vi "reg_visu OPC.vi"(7 "name":string="GM10", 9 "stop":bool, 10 "connect (T)":bool=TRUE) -> (0 "error out":errorcluster, 5 "This VI":refnum<vi>)   [LabVIEW 2019]
uses:
  Heating/ctl/Z_OnSwitch/Z_OnSwitch.xctl
  Heating/ctl/Z_ind_heating.ctl
  Heating/ctl/Z_Hswitch/Z_Hswitch.xctl
  ctl/Y/Y.xctl
  Heating/ctl/Z_State.ctl
  Heating/ctl/Y_state.ctl
  <vilib>/OPCUA/controls/OPC UA StatusCode.ctl
  Heating/ctl/ZY_state.ctl
  Heating/ctl/Z.ctl
  Heating/ctl/Y_source.ctl
  Heating/ctl/ZM_State.ctl
  Heating/ctl/Y.ctl
  Inputs/Ctl/Parameter State.ctl
  Alarms/Ctl/ALR_Status.ctl
  Heating/ctl/ZY_state_OPC.ctl
  <vilib>/OPCUA/controls/Write Variant Request.ctl
  <vilib>/OPCUA/controls/NodeId.ctl
  <vilib>/OPCUA/controls/Write Status.ctl
  08a30d42-25e3-4a58-beca-1d562a75ea40.vi
  fbc51cc2-a17d-4d51-90ca-ef1d5e9adb43.vi
  81bac83f-5a8a-4521-9bb9-45d0222ee4c6.vi
  3276b797-77fd-4487-96b2-8bfe15282525.vi
  45230f51-ed9d-4592-a49a-e0edfe92ddd1.vi
  <vilib>/NI/AMC/Read Termination Message.vi
  <vilib>/NI/AMC/Create Single Message.vi
  <vilib>/NI/AMC/Update Message Routing Info.vi
  Counter/Generator simplified.vi
  <vilib>/NI/AMC/Globals.vi
  <vilib>/NI/AMC/Send Message.vi
  Heating/Global stop.vi
  <vilib>/OPCUA/client/Multiple Read String.vi
  <vilib>/JDP Science/JSONtext/JSON text to Variant.vi
  <vilib>/OPCUA/client/Multiple Write Variant.vi
  Heating/Heating.lvlib
  <vilib>/OPCUA/NI OPC UA Client.lvlib
  OPC/OPC addons.lvlib
  Inputs/Inputs.lvlib
  <vilib>/NI/AMC/AMC.lvlib
  Alarms/Alarms.lvlib
panel:
  out "PV":dbl(slide) scale=0.0..10.0
  in  "Scale max":dbl=1.0 format="%#_13g"
  in  "name 4":string="Осн."
  in  "Unit":enum16{"l/h", "m3/h"}(ring)
  in  "name 3":string="Осн."
  in  "t":dbl=10.5 caption="сек."
  in  "alarm val":dbl=3.01 caption="m3/h"
  in  "auto":dbl=15.888 caption="Зависимый"
  in  "k":dbl=1.459 caption="Коэфф"
  in  "Y_SP":cluster{dbl, dbl, dbl}(xcontrol)
  in  "message name":string="AI redefine"
  out "status":string
  in  "process":bool
  in  "state variables":cluster{"CurrentFile":path}
  in  "security policy":T1
  out "JSON string":string
  in  "JSON":string
  in  "Write controls":bool
  out "T stage":dbl format="%<%M:%S>t"
  in  "ALRL1_reset":bool
  in  "ALRL2_reset":bool
  out "Z3 ind":T2
  in  "Z_OnSwitch":bool(xcontrol)
  in  "Z_Hswitch":bool(xcontrol)
  out "Z5 State":string
  # "Время установки"
  # "Аварийный"
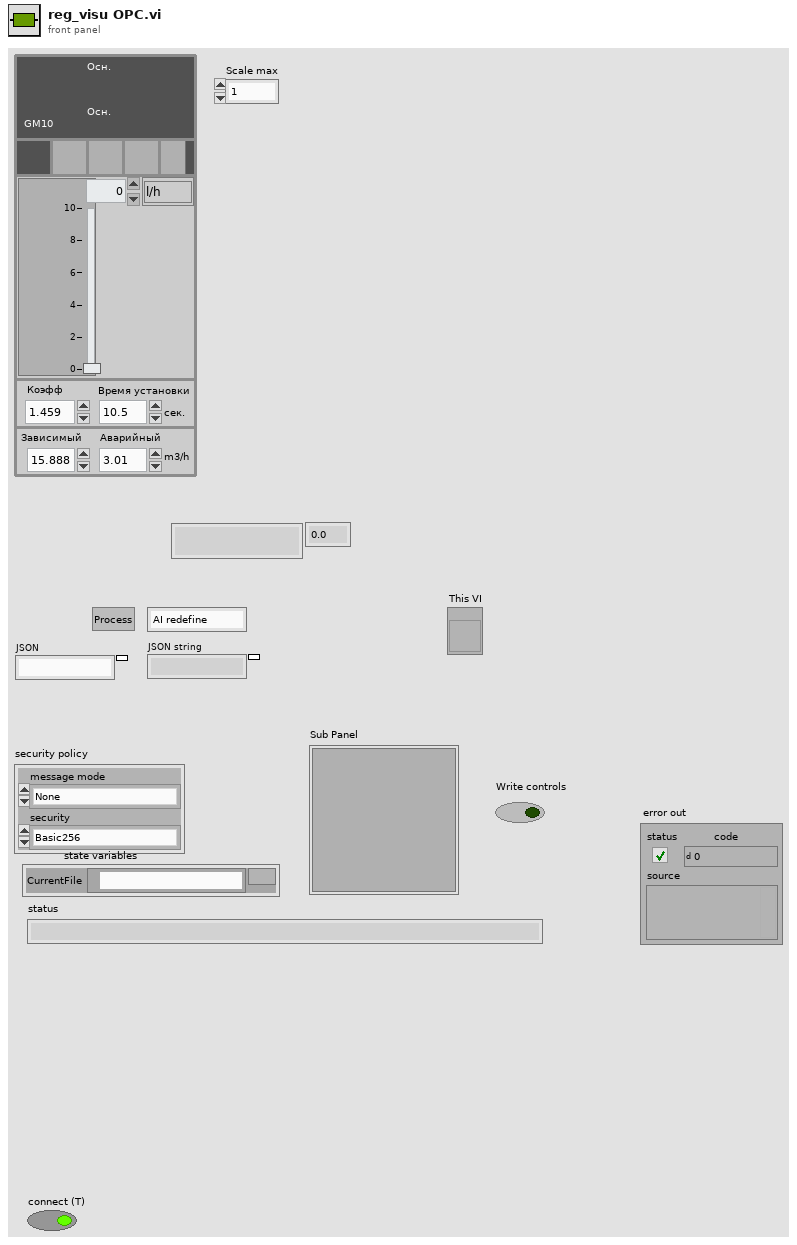
[diagram p1: front panel]
types:
  T1 = cluster{"message mode":enum16{"None", "Sign", "Sign and Encrypt"}, "security":enum16{"Basic256", "Basic128Rsa15"}}
  T2 = typedef "Heating.lvlib/Z_ind_heating.ctl" = u16
  T3 = typedef "AMC.lvlib/Message Queue.ctl" = refnum<queue>
  T4 = typedef "Write Variant Request.ctl" = cluster{"node ID":T5, "value":variant, "timestamp (current time)":timestamp, "node status":T6}
  T5 = typedef "NodeId.ctl" = string
  T6 = typedef "Write Status.ctl" = u32
  T7 = typedef "OPC UA Client Refnum.ctl" = refnum<k21>
  T8 = typedef "Subscription ID.ctl" = u32
  T9 = typedef "Heating.lvlib/Y_source.ctl" = enum8{"initialize", "local disabled", "local hand", "hand", "auto", "dist"}
  T10 = cluster{"connect":bool, "SP_Source":T9, "SP_Set":dbl, "SP":dbl}
  T11 = typedef "Heating.lvlib/Z_State.ctl" = enum8{"initialization", "alarm", "disabled", "not ready", "stop ready", "reserv", "switched off", "reserv2", "switched on", "check", "on min", "decrease out", "on", "increase out", "on max"}
  T12 = cluster{"connect":bool, "Z_Source":T9, "Z_State_heating":T11}
  T13 = typedef "Heating.lvlib/ZM_State.ctl" = enum8{"initialization", "stop", "start_cmd", "contactor_on_cmd", "heating", "on", "stop_cmd", "power_down", "contactor_off_cmd", "cooling", "restart_delay"}
  T14 = typedef "Heating.lvlib/ZY_state_OPC.ctl" = cluster{"Z":cluster{"Z_Source":u8, "Z_SetState":u8, "Z_State":u8, "Z_State_T":u32, "ZM_State":u8, "ZM_State_T":u32, "ALR  L1":bool, "ALR  L2":bool, "HH_run":i32}, "Y":cluster{"Y_Source":u8, "Y_SetState":u8, "SP_Set":dbl, "SP":dbl, "PV":dbl, "Y":dbl, "Y_State":cluster{"code":i32, "visible":bool, "color":u32}, "YB":bool}, "ALR_Status":cluster{"status":bool, "code":i32, "level":i32}[]}
  T15 = cluster{"Z_HSw":u32, "Z_HSetState":u32, "Y_HSw":u32, "Y_HSetState":u32, "SP":dbl, "Y_H":dbl, "Reset_ALR":bool}
  T16 = typedef "Heating.lvlib/Y_state.ctl" = enum8{"initialize", "alarm", "min", "stop", "hand", "auto", "max"}
  T17 = typedef "Heating.lvlib/ZY_state.ctl" = cluster{"Z":T18, "Y":T19, "ALR_Status":T21[]}
  T18 = typedef "Heating.lvlib/Z.ctl" = cluster{"Z_Source":T9, "Z_SetState":T11, "Z_State":T11, "Z_State_T":u32, "ZM_State":T13, "ZM_State_T":u32, "ALR  L1":bool, "ALR  L2":bool, "HH_run":i32}
  T19 = typedef "Heating.lvlib/Y.ctl" = cluster{"Y_Source":T9, "Y_SetState":T16, "SP_Set":dbl, "SP":dbl, "PV":dbl, "Y":dbl, "Y_State":T20, "YB":bool}
  T20 = typedef "Inputs.lvlib/Parameter State.ctl" = cluster{"code":i32, "visible":bool, "color":u32, "source":string}
  T21 = typedef "Alarms.lvlib/ALR_Status.ctl" = cluster{"status":bool, "code":i32, "level":i32, "source":string}
  T22 = typedef "OPC UA StatusCode.ctl" = u32
  T23 = enum32{"Invalid Status", "Unconnected", "Active", "Idle", "Error", "Connecting"}
  T24 = cluster{"node ID":T5, "value ":string, "timestamp":timestamp, "status":T22}[]
  T25 = typedef "LVDataSocketStatusTypeDef.ctl" = cluster{"Code":enum32{"Invalid Status", "Unconnected", "Active", "Idle", "Error", "Connecting"}, "Text":string}
  T26 = cluster{"node ID":T5, "value ":string, "timestamp":timestamp, "status":T22}
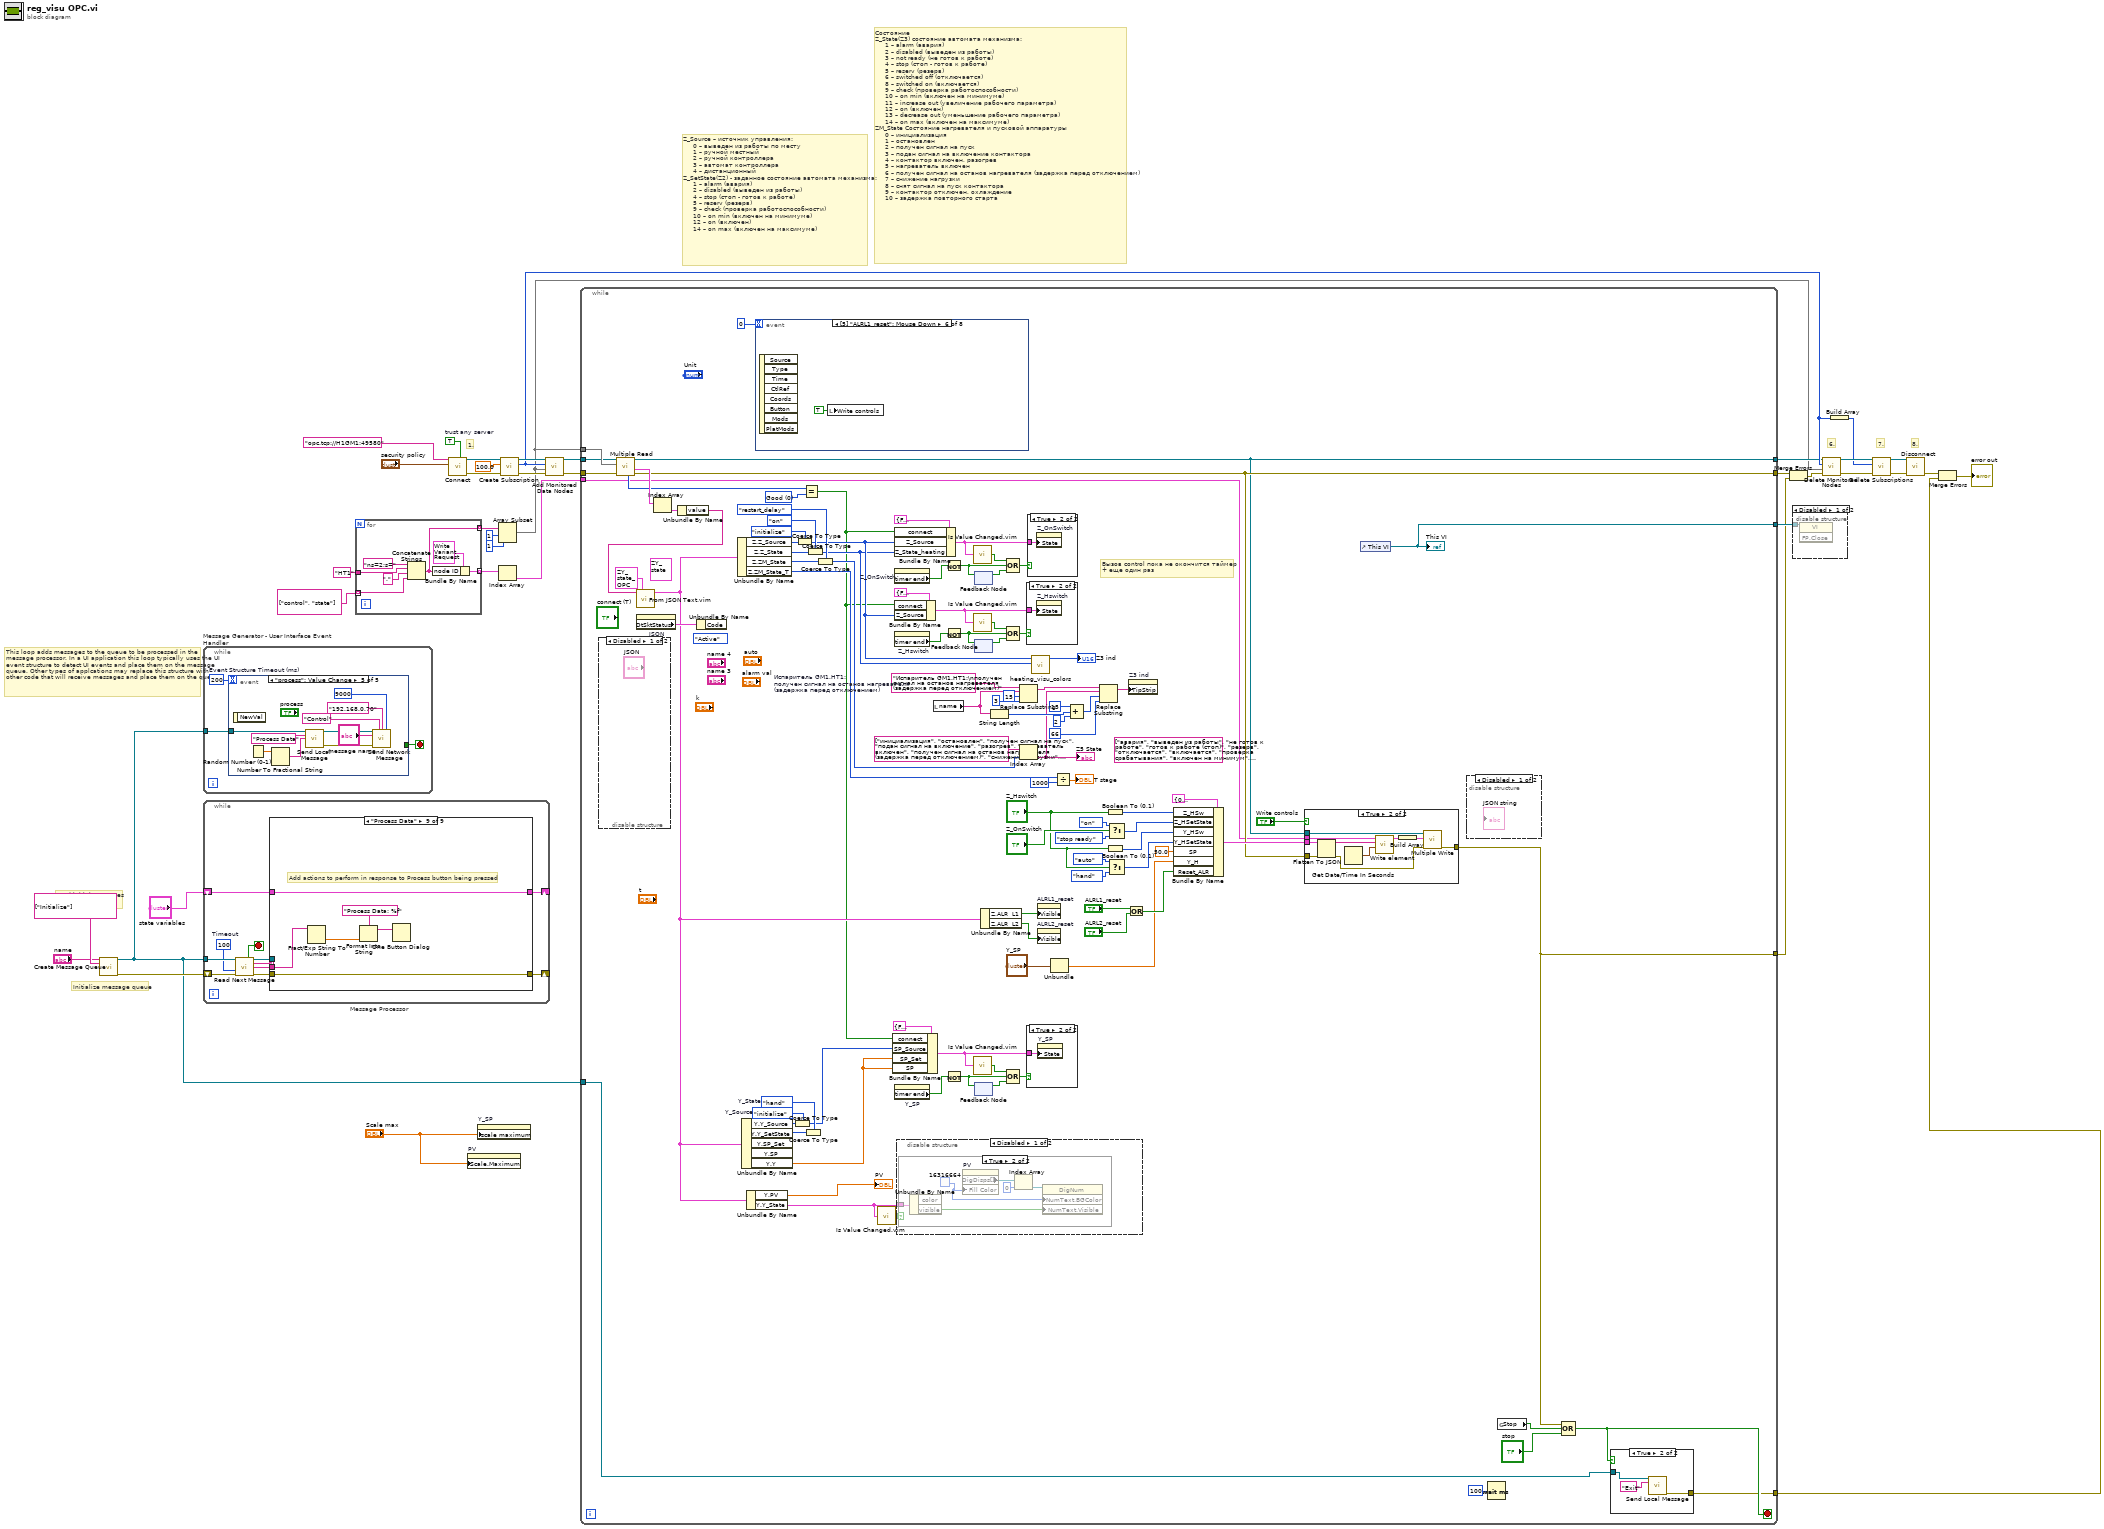
[diagram p0: block diagram]
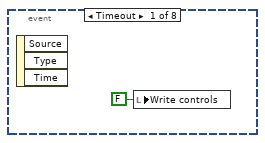
[diagram p9: hidden frame]
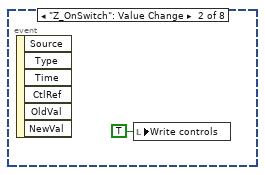
[diagram p10: hidden frame]
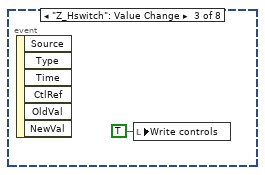
[diagram p11: hidden frame]
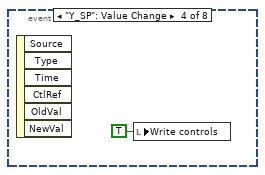
[diagram p12: hidden frame]
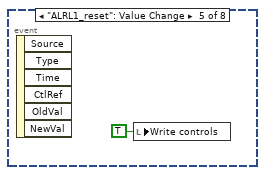
[diagram p13: hidden frame]
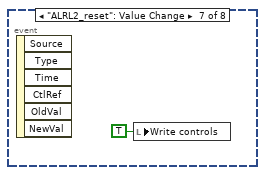
[diagram p14: hidden frame]
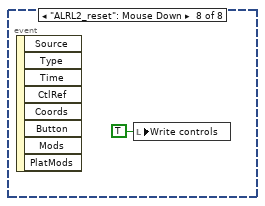
[diagram p15: hidden frame]
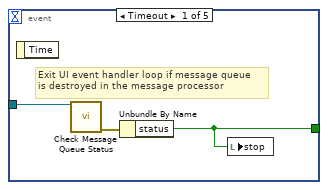
[diagram p19: hidden frame]
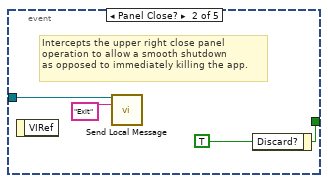
[diagram p20: hidden frame]
diagram:
  w31 = TRUE  # trust any server
  # "This loop adds messages to the queue to be processed in the message processor. In a UI application this loop typically uses the UI event structure to detect UI events and place them on the message queue. Other types of applcations may replace this structure with other code that will receive messages and place them on the queue."
  # "Initialize message queue"
  # "Load initial messages\non the queue"
  # "7."
  # "8."
  # "6."
  # "1."
  # "Состояние\nZ_State(Z3) состояние автомата механизма:\n     1 – alarm (авария)\n     2 – disabled (выведен из работы)\n     3 – not ready (не готов к работе)\n     4 – stop (стоп - готов к работе)\n     5 – reserv (резерв)\n     6 – switched off (отключается)\n     8 – switched on (включается)\n     9 – check (проверка работоспособности)\n     10 – on min (включен на минимуме)\n     11 – increase out (увеличение рабочего параметра)\n     12 – on (включен)\n     13 – decrease out (уменьшение рабочего параметра)\n     14 – on max (включен на максимуме)\nZM_State Состояние нагревателя и пусковой аппаратуры\n     0 – инициализация\n     1 – остановлен\n     2 – получен сигнал на пуск\n     3 – подан сигнал на включение контактора\n     4 – контактор включен, разогрев\n     5 – нагреватель включен\n     6 – получен сигнал на останов нагревателя (задержка перед отключением)\n     7 – снижение нагрузки\n     8 – снят сигнал на пуск контактора\n     9 – контактор отключен, охлаждение\n     10 – задержка повторного старта"
  # "Z_Source – источник управления:\n     0 – выведен из работы по месту\n     1 – ручной местный\n     2 – ручной контроллера\n     3 – автомат контроллера\n     4 – дистанционный\nZ_SetState(Z2) - заданное состояние автомата механизма:\n     1 – alarm (авария)\n     2 – disabled (выведен из работы)\n     4 – stop (стоп - готов к работе)\n     5 – reserv (резерв)\n     9 – check (проверка работоспособности)\n     10 – on min (включен на минимуме)\n     12 – on (включен)\n     14 – on max (включен на максимуме)"
  n1 = call <vilib>:"Create Message Queue.vi"("message queue name"="name", "initial message names"=string[] ["Initialize"]) -> ("message queue out"=w6:T3, "error out"=w8:errorcluster)  [unwired: 12 in]
  n2 = while "Message Generator - User Interface Event Handler" {
    tunnel: w6 -> [w39]
    stop <- w40 stop-if-true
    w41 = 200  # Event Structure Timeout (ms)
    n3 = event shown="[4] \"process\": Value Change" {
      selector: _ -> [_ _ _ _ _]
      dyn-events: _ -> [_ _ _ _ _]
      timeout: w41 -> [_ _ _ _ _]
      tunnel: [w42 w47 TRUE ("Discard?") _ _] -> w40
      tunnel: w39 -> [w43 w45 w48 w51 w62]
      event Timeout {
        # "Exit UI event handler loop if message queue\nis destroyed in the message processor"
        n4 = event-data() -> ()  [unwired: 2 out]
        n5 = call <vilib>:"Check Message Queue Status.vi"("message queue in"=w43) -> ("error out"=w44:errorcluster)  [unwired: 10 in, 4 out]
        n6 = Unbundle By Name(w44) -> ("status"=w42:bool)
        n7 = local write "stop"(w42) -> ()
      }
      event Panel Close? {
        w47 = TRUE ("Discard?")
        # "Intercepts the upper right close panel\noperation to allow a smooth shutdown\nas opposed to immediately killing the app."
        n8 = event-data() -> ()  [unwired: 2 out]
        n9 = call <vilib>:"Send Local Message.vi"("message queue in"=w45, "message name"="Exit") -> ()  [unwired: 11 in, 3 out]
        n10 = event-data("Discard?"=w47) -> ()  [unwired: 1 in, 1 out]
      }
      event "stop": Value Change {
        # "Exit the application\n>> Stop this message generator loop"
        n11 = event-data() -> ()  [unwired: 7 out]
        n12 = call <vilib>:"Send Local Message.vi"("message queue in"=w48, "message name"="Exit") -> ()  [unwired: 11 in, 3 out]
      }
      event Menu Selection (User) {
        # "Add run-time menu items to the message\nqueue. The message handler case names must match the menu ItemTag names."
        n13 = event-data() -> ("ItemTag"=w52:string)  [unwired: 1 out]
        n14 = call <vilib>:"Send Local Message.vi"("message queue in"=w51, "message name"=w52) -> ()  [unwired: 11 in, 3 out]
      }
      event "process": Value Change {
        n15 = event-data() -> ()  [unwired: 2 out]
        n16 = Random Number (0-1)() -> (number: 0 to 1=w59:dbl)
        n17 = Number To Fractional String(number=w59) -> (F-format string=w60:string)  [unwired: 3 out]
        n18 = call <vilib>:"Send Local Message.vi"("message queue in"=w62, "message name"="Process Data", "message value"=w60) -> ("message queue out"=w58:T3, "error out"=w54:errorcluster)  [unwired: 10 in, 1 out]
        n19 = call <vilib>:"Send Network Message.vi"("message queue in"=w58, "receiver process"="Control", "receiver host"="192.168.0.70", "receiver port (0)"=u16 9000, "message name"="message name", "error in"=w54) -> ()  [unwired: 7 in, 3 out]
      }
    }
  }
  n20 = while "Message Processor" {
    shift-left: w8 -> [w67]
    shift-right: [w71] -> _
    tunnel: w6 -> [w68]
    shift-left: "state variables" -> [w73]
    shift-right: [w72] -> _
    stop <- w70 stop-if-true
    w63 = 100  # Timeout
    n21 = call <vilib>:"Read Next Message.vi"("message queue in"=w68, "timeout (1 ms)"=w63, "error in"=w67) -> ("exit process?"=w70:bool, "message queue out"=w69:T3, "message name"=w65:string, "message value"=w64:string, "error out"=w66:errorcluster)  [unwired: 5 in, 3 out]
    n22 = case shown="\"Process Data\"" w65 {
      selector: w65 -> [_ _ w85 _ _ _ _ _ _]
      tunnel: [w75 w82 w87 w92 w94 w96 w101 w103 w108] -> w72
      tunnel: w73 -> [w75 w82 w87 w92 w94 w96 w101 w103 w108]
      tunnel: w69 -> [_ _ _ w90 _ _ w98 _ _]
      tunnel: w66 -> [w74 w81 w86 w88 w93 w95 w99 w102 w109]
      tunnel: [w74 w81 w86 errorcluster {"status"=FALSE, "code"=0, "source"=""} ("error out") w93 w95 w97 w102 w109] -> w71
      tunnel: w64 -> [_ _ _ _ _ _ _ _ w107]
      frame "---------- Framework Operations ----------" {
        # "Dummy case to add a seperator in the Case Structure menu"
      }
      frame "", "Idle" {
        # "Update the front panel"
        # "Idle Case - this case is called after a Timeout on the Get Next Message from Queue VI, if no new messages are present on the queue. This case can be used for housekeeping tasks such as updating the UI."
        n23 = Get Date/Time String(want seconds? (F)=TRUE) -> (date string=w80:string, time string=w79:string)  [unwired: 2 out]
        n24 = Concatenate Strings(w80, " " ("string"), w79) -> (→"status":string)
      }
      frame "Missing Message Handler", Default {
        # "Call this case if a message is received that is not handled \nby any other case. Typically this is a programming error\nas a result of a typo or unhandled message/missing message handler."
        n25 = Format Into String(format string="DevError: Missing message handler for '%s\" message." ("message"), w85) -> (resulting string=w83:string)  [unwired: 2 in, 1 out]
        n26 = One Button Dialog(message=w83) -> ()  [unwired: 2 out]
      }
      frame "Error" {
        # "Proceed to Exit - Remove this if it is\nnot appropriate for the General Error case"
        # "General Error Case - this case is called if an error is passed using the error cluster below. Typically most new errors should be handed in each individual case and not passed in the rror cluster. If necessary a custom error handler case should be added and called from other cases."
        n27 = call <vilib>:"Simple Error Handler.vi"("error in (no error)"=w88) -> ()  [unwired: 1 in, 8 out]
        n28 = call <vilib>:"Send Local Message.vi"("message queue in"=w90, "message name"="Exit") -> ()  [unwired: 11 in, 3 out]
      }
      frame "---------- Generic Operations ----------" {
        # "Dummy case to add a seperator in the Case Structure menu"
      }
      frame "Initialize" {
        # "Initialize the state variables and user interface"
      }
      frame "Exit" {
        # "Destroy message queue >> this will halt the UI event handler loop"
        # "Stop the VI\n>> Perform any cleanup tasks in this message case.\n>> Clear display before closing."
        n29 = call <vilib>:"Destroy Message Queue.vi"("message queue in"=w98, "error in"=w99) -> ("error out"=w97:errorcluster)  [unwired: 11 in, 2 out]
        n30 = local write "status"("" ("Status")) -> ()
      }
      frame "---------- Application Operations ----------" {
        # "Dummy case to add a seperator in the Case Structure menu"
      }
      frame "Process Data" {
        # "Add actions to perform in response to Process button being pressed"
        n31 = Fract/Exp String To Number(string=w107) -> (number=w106:dbl)  [unwired: 4 out]
        n32 = Format Into String(format string="Process Data: %f" ("message"), w106) -> (resulting string=w104:string)  [unwired: 2 in, 1 out]
        n33 = One Button Dialog(message=w104) -> ()  [unwired: 2 out]
      }
    }
  }
  n34 = for {
    tunnel: string[] ["control", "state"] -> [w110] mode=indexing
    tunnel: "HT1" ("Folder Name") -> [w116]
    tunnel: [w113] -> w20 mode=indexing
    tunnel: [w112] -> w16 mode=indexing
    n35 = Concatenate Strings("ns=2;s=" ("string"), w116, "." ("string"), w110) -> (w113:string)
    n36 = Bundle By Name(cluster=T4 {"node ID"="", "value"=variant, "timestamp (current time)"=timestamp(0 s since 1904-01-01), "node status"=0} ("request"), "node ID"=w113) -> (w112:T4)
  }
  n37 = call <vilib>:"Connect.vi"("trust any server (F)"=w31, "security policy"="security policy", "server endpoint URL"="opc.tcp://H1GM1:49580" ("server endpoint URL 2")) -> ("error out"=w34:errorcluster, "OPC UA client refnum out"=w35:T7)  [unwired: 6 in, 1 out]
  n38 = property on="PV" class="Slide (strict)"("Scale.Maximum"="Scale max") -> ()  [unwired: 2 in, 2 out]
  n39 = property on="Y_SP" class="Y (strict)"("scale maximum"="Scale max") -> ()  [unwired: 2 in, 2 out]
  n40 = Array Subset(array=w20, index=1, length=1) -> (w10:string[])
  n41 = Index Array(array=w16) -> (element=w14:T4)  [unwired: 1 in]
  n42 = call <vilib>:"Create Subscription.vi"("error in (no error)"=w34, "publishing interval (1000 ms)"=100.0 ("update rate (1000 ms)"), "OPC UA client refnum in"=w35) -> ("error out"=w36:errorcluster, "subscription ID out"=w24:T8, "OPC UA client refnum out"=w37:T7)  [unwired: 4 in, 2 out]
  n43 = call <vilib>:"Add Monitored Data Nodes.vi"("error in (no error)"=w36, "node IDs"=w10, "subscription ID in"=w24, "OPC UA client refnum in"=w37) -> ("error out"=w17:errorcluster, "OPC UA client refnum out"=w18:T7)  [unwired: 4 in, 2 out]
  n44 = while {
    tunnel: [w180] -> w38
    tunnel: w18 -> [w169]
    tunnel: w17 -> [w176]
    tunnel: w14 -> [w168]
    tunnel: [w167] -> w13
    tunnel: [w169] -> w12
    tunnel: [w171] -> w11
    tunnel: w10 -> [w175]
    tunnel: w6 -> [w165]
    tunnel: [w164] -> w4
    stop <- w166 stop-if-true
    w153 = Y_state."hand"  # Y_State
    w154 = Y_source."initialize"  # Y_Source
    (unwired) T17 {"Z"={"Z_Source"=enum."initialize", "Z_SetState"=enum."initialization", "Z_State"=enum."initialization", "Z_State_T"=0, "ZM_State"=enum."initialization", "ZM_State_T"=0, "ALR  L1"=FALSE, "ALR  L2"=FALSE, "HH_run"=0}, "Y"={"Y_Source"=enum."initialize", "Y_SetState"=enum."initialize", "SP_Set"=0.0, "SP"=0.0, "PV"=0.0, "Y"=0.0, "Y_State"={"code"=0, "visible"=FALSE, "color"=0, "source"=""}, "YB"=FALSE}, "ALR_Status"=[]} ("HT1_state")
    w173 = T22 0 items=["Good"=0, "Good_SubscriptionTransferred"=2949120, "Good_CompletesAsynchronously"=3014656, "Good_Overload"=3080192, "Good_Clamped"=3145728, "Good_LocalOverride"=9830400, "Good_EntryInserted"=10616832, "Good_EntryReplaced"=10682368, "Good_NoData"=10813440, "Good_MoreData"=10878976, "Good_CommunicationEvent"=10944512, "Good_ShutdownEvent"=11010048, "Good_CallAgain"=11075584, "Good_NonCriticalTimeout"=11141120, "Good_ResultsMayBeIncomplete"=12189696, "Good_DataIgnored"=14221312, "Uncertain"=1073741824, "Uncertain_ReferenceOutOfServer"=1080819712, "Uncertain_NoCommunicationLastUsableValue"=1083113472, "Uncertain_LastUsableValue"=1083179008, "Uncertain_SubstituteValue"=1083244544, "Uncertain_InitialValue"=1083310080, "Uncertain_SensorNotAccurate"=1083375616, "Uncertain_EngineeringUnitsExceeded"=1083441152, "Uncertain_SubNormal"=1083506688, "Uncertain_DataSubNormal"=1084489728, "Uncertain_ReferenceNotDeleted"=1086062592, "Uncertain_NotAllNodesAvailable"=1086324736, "Bad"=2147483648, "Bad_UnexpectedError"=2147549184, "Bad_InternalError"=2147614720, "Bad_OutOfMemory"=2147680256, "Bad_ResourceUnavailable"=2147745792, "Bad_CommunicationError"=2147811328, "Bad_EncodingError"=2147876864, "Bad_DecodingError"=2147942400, "Bad_EncodingLimitsExceeded"=2148007936, "Bad_UnknownResponse"=2148073472, "Bad_Timeout"=2148139008, "Bad_ServiceUnsupported"=2148204544, "Bad_Shutdown"=2148270080, "Bad_ServerNotConnected"=2148335616, "Bad_ServerHalted"=2148401152, "Bad_NothingToDo"=2148466688, "Bad_TooManyOperations"=2148532224, "Bad_DataTypeIdUnknown"=2148597760, "Bad_CertificateInvalid"=2148663296, "Bad_SecurityChecksFailed"=2148728832, "Bad_CertificateTimeInvalid"=2148794368, "Bad_CertificateIssuerTimeInvalid"=2148859904, "Bad_CertificateHostNameInvalid"=2148925440, "Bad_CertificateUriInvalid"=2148990976, "Bad_CertificateUseNotAllowed"=2149056512, "Bad_CertificateIssuerUseNotAllowed"=2149122048, "Bad_CertificateUntrusted"=2149187584, "Bad_CertificateRevocationUnknown"=2149253120, "Bad_CertificateIssuerRevocationUnknown"=2149318656, "Bad_CertificateRevoked"=2149384192, "Bad_CertificateIssuerRevoked"=2149449728, "Bad_UserAccessDenied"=2149515264, "Bad_IdentityTokenInvalid"=2149580800, "Bad_IdentityTokenRejected"=2149646336, "Bad_SecureChannelIdInvalid"=2149711872, "Bad_InvalidTimestamp"=2149777408, "Bad_NonceInvalid"=2149842944, "Bad_SessionIdInvalid"=2149908480, "Bad_SessionClosed"=2149974016, "Bad_SessionNotActivated"=2150039552, "Bad_SubscriptionIdInvalid"=2150105088, "Bad_RequestHeaderInvalid"=2150236160, "Bad_TimestampsToReturnInvalid"=2150301696, "Bad_RequestCancelledByClient"=2150367232, "Bad_NoCommunication"=2150694912, "Bad_WaitingForInitialData"=2150760448, "Bad_NodeIdInvalid"=2150825984, "Bad_NodeIdUnknown"=2150891520, "Bad_AttributeIdInvalid"=2150957056, "Bad_IndexRangeInvalid"=2151022592, "Bad_IndexRangeNoData"=2151088128, "Bad_DataEncodingInvalid"=2151153664, "Bad_DataEncodingUnsupported"=2151219200, "Bad_NotReadable"=2151284736, "Bad_NotWritable"=2151350272, "Bad_OutOfRange"=2151415808, "Bad_NotSupported"=2151481344, "Bad_NotFound"=2151546880, "Bad_ObjectDeleted"=2151612416, "Bad_NotImplemented"=2151677952, "Bad_MonitoringModeInvalid"=2151743488, "Bad_MonitoredItemIdInvalid"=2151809024, "Bad_MonitoredItemFilterInvalid"=2151874560, "Bad_MonitoredItemFilterUnsupported"=2151940096, "Bad_FilterNotAllowed"=2152005632, "Bad_StructureMissing"=2152071168, "Bad_EventFilterInvalid"=2152136704, "Bad_ContentFilterInvalid"=2152202240, "Bad_FilterOperandInvalid"=2152267776, "Bad_ContinuationPointInvalid"=2152333312, "Bad_NoContinuationPoints"=2152398848, "Bad_ReferenceTypeIdInvalid"=2152464384, "Bad_BrowseDirectionInvalid"=2152529920, "Bad_NodeNotInView"=2152595456, "Bad_ServerUriInvalid"=2152660992, "Bad_ServerNameMissing"=2152726528, "Bad_DiscoveryUrlMissing"=2152792064, "Bad_SempahoreFileMissing"=2152857600, "Bad_RequestTypeInvalid"=2152923136, "Bad_SecurityModeRejected"=2152988672, "Bad_SecurityPolicyRejected"=2153054208, "Bad_TooManySessions"=2153119744, "Bad_UserSignatureInvalid"=2153185280, "Bad_ApplicationSignatureInvalid"=2153250816, "Bad_NoValidCertificates"=2153316352, "Bad_RequestCancelledByRequest"=2153381888, "Bad_ParentNodeIdInvalid"=2153447424, "Bad_ReferenceNotAllowed"=2153512960, "Bad_NodeIdRejected"=2153578496, "Bad_NodeIdExists"=2153644032, "Bad_NodeClassInvalid"=2153709568, "Bad_BrowseNameInvalid"=2153775104, "Bad_BrowseNameDuplicated"=2153840640, "Bad_NodeAttributesInvalid"=2153906176, "Bad_TypeDefinitionInvalid"=2153971712, "Bad_SourceNodeIdInvalid"=2154037248, "Bad_TargetNodeIdInvalid"=2154102784, "Bad_DuplicateReferenceNotAllowed"=2154168320, "Bad_InvalidSelfReference"=2154233856, "Bad_ReferenceLocalOnly"=2154299392, "Bad_NoDeleteRights"=2154364928, "Bad_ServerIndexInvalid"=2154430464, "Bad_ViewIdUnknown"=2154496000, "Bad_TooManyMatches"=2154627072, "Bad_QueryTooComplex"=2154692608, "Bad_NoMatch"=2154758144, "Bad_MaxAgeInvalid"=2154823680, "Bad_HistoryOperationInvalid"=2154889216, "Bad_HistoryOperationUnsupported"=2154954752, "Bad_WriteNotSupported"=2155020288, "Bad_TypeMismatch"=2155085824, "Bad_MethodInvalid"=2155151360, "Bad_ArgumentsMissing"=2155216896, "Bad_TooManySubscriptions"=2155282432, "Bad_TooManyPublishRequests"=2155347968, "Bad_NoSubscription"=2155413504, "Bad_SequenceNumberUnknown"=2155479040, "Bad_MessageNotAvailable"=2155544576, "Bad_InsufficientClientProfile"=2155610112, "Bad_TcpServerTooBusy"=2155675648, "Bad_TcpMessageTypeInvalid"=2155741184, "Bad_TcpSecureChannelUnknown"=2155806720, "Bad_TcpMessageTooLarge"=2155872256, "Bad_TcpNotEnoughResources"=2155937792, "Bad_TcpInternalError"=2156003328, "Bad_TcpEndpointUrlInvalid"=2156068864, "Bad_RequestInterrupted"=2156134400, "Bad_RequestTimeout"=2156199936, "Bad_SecureChannelClosed"=2156265472, "Bad_SecureChannelTokenUnknown"=2156331008, "Bad_SequenceNumberInvalid"=2156396544, "Bad_ConfigurationError"=2156462080, "Bad_NotConnected"=2156527616, "Bad_DeviceFailure"=2156593152, "Bad_SensorFailure"=2156658688, "Bad_OutOfService"=2156724224, "Bad_DeadbandFilterInvalid"=2156789760, "Bad_RefreshInProgress"=2157379584, "Bad_ConditionAlreadyDisabled"=2157445120, "Bad_ConditionDisabled"=2157510656, "Bad_EventIdUnknown"=2157576192, "Bad_NoData"=2157641728, "Bad_DataLost"=2157772800, "Bad_DataUnavailable"=2157838336, "Bad_EntryExists"=2157903872, "Bad_NoEntryExists"=2157969408, "Bad_TimestampNotSupported"=2158034944, "Bad_InvalidArgument"=2158690304, "Bad_ConnectionRejected"=2158755840, "Bad_Disconnect"=2158821376, "Bad_ConnectionClosed"=2158886912, "Bad_InvalidState"=2158952448, "Bad_EndOfStream"=2159017984, "Bad_NoDataAvailable"=2159083520, "Bad_WaitingForResponse"=2159149056, "Bad_OperationAbandoned"=2159214592, "Bad_ExpectedStreamToBlock"=2159280128, "Bad_WouldBlock"=2159345664, "Bad_SyntaxError"=2159411200, "Bad_MaxConnectionsReached"=2159476736, "Bad_RequestTooLarge"=2159542272, "Bad_ResponseTooLarge"=2159607808, "Bad_EventNotAcknowledgeable"=2159738880, "Bad_InvalidTimestampArgument"=2159869952, "Bad_ProtocolVersionUnsupported"=2159935488, "Bad_StateNotActive"=2160001024, "Bad_FilterOperatorInvalid"=2160132096, "Bad_FilterOperatorUnsupported"=2160197632, "Bad_FilterOperandCountMismatch"=2160263168, "Bad_FilterElementInvalid"=2160328704, "Bad_FilterLiteralInvalid"=2160394240, "Bad_IdentityChangeNotSupported"=2160459776, "Bad_NotTypeDefinition"=2160590848, "Bad_ViewTimestampInvalid"=2160656384, "Bad_ViewParameterMismatch"=2160721920, "Bad_ViewVersionInvalid"=2160787456, "Bad_ConditionAlreadyEnabled"=2160852992, "Bad_DialogNotActive"=2160918528, "Bad_DialogResponseInvalid"=2160984064, "Bad_ConditionBranchAlreadyAcked"=2161049600, "Bad_ConditionBranchAlreadyConfirmed"=2161115136, "Bad_ConditionAlreadyShelved"=2161180672, "Bad_ConditionNotShelved"=2161246208, "Bad_ShelvingTimeOutOfRange"=2161311744, "Bad_AggregateListMismatch"=2161377280, "Bad_AggregateNotSupported"=2161442816, "Bad_AggregateInvalidInputs"=2161508352, "Bad_BoundNotFound"=2161573888, "Bad_BoundNotSupported"=2161639424, "Bad_AggregateConfigurationRejected"=2161770496, "Bad_TooManyMonitoredItems"=2161836032] ("y")
    (unwired) T23."Active" ("Code")
    (unwired) string[] ["авария", "выведен из работы", "не готов к работе", "готов к работе (стоп)", "резерв", "отключается", "включается", "проверка срабатывания", "включен на минимум", "увеличение произв", "включен", "уменьшение произв", "включен на максимум"]
    w213 = "Испаритель GM1.HT1:\nполучен сигнал на останов нагревателя (задержка перед отключением)"  # Испаритель GM1.HT1: получен сигнал на останов нагревателя (задержка перед отключением)
    # "Вызов control пока не окончится таймер\n+ еще один раз"
    n45 = disable-structure shown="Disabled" {
      frame Disabled {
      }
      frame Enabled {
      }
    }
    n46 = call-poly <vilib>:"Multiple Read.vi"("error in (no error)"=w176, "node IDs"=w175, "OPC UA client refnum in"=w169) -> ("error out"=w171:errorcluster, "results"=w178:T24, "service status"=w174:T22)  [unwired: 5 in, 1 out]
    n47 = property on="JSON" class="Str"() -> ("DtSktStatus"=w181:T25)  [unwired: 2 in, 2 out]
    n48 = Index Array(array=w178) -> (element=w177:T26)  [unwired: 1 in]
    n49 = Unbundle By Name(w177) -> ("value"=w170:string)
    n50 = call "From JSON Text.vim"("Data Type and Default Value"=T14 {"Z"={"Z_Source"=0, "Z_SetState"=0, "Z_State"=0, "Z_State_T"=0, "ZM_State"=0, "ZM_State_T"=0, "ALR  L1"=FALSE, "ALR  L2"=FALSE, "HH_run"=0}, "Y"={"Y_Source"=0, "Y_SetState"=0, "SP_Set"=0.0, "SP"=0.0, "PV"=0.0, "Y"=0.0, "Y_State"={"code"=0, "visible"=FALSE, "color"=0}, "YB"=FALSE}, "ALR_Status"=[]} ("ZY_State"), "JSON"=w170) -> ("Data out"=w133:T14)  [unwired: 8 in, 1 out]
    n51 = Unbundle By Name(w181) -> ()  [unwired: 1 out]
    n52 = Unbundle By Name(w133) -> ("Z.Z_Source"=w160:u8, "Z.Z_State"=w193:u8, "Z.ZM_State"=w188:u8, "Z.ZM_State_T"=w195:u32)
    n53 = Unbundle By Name(w133) -> ("Y.Y_Source"=w159:u8, "Y.Y_SetState"=w194:u8, "Y.Y"=w122:dbl)  [unwired: 2 out]
    n54 = Unbundle By Name(w133) -> ("Y.PV"=→"PV":dbl, "Y.Y_State"=w132:cluster{"code":i32, "visible":bool, "color":u32})
    n55 = event shown="[5] \"ALRL1_reset\": Mouse Down" {
      selector: _ -> [_ _ _ _ _ _ _ _]
      dyn-events: _ -> [_ _ _ _ _ _ _ _]
      timeout: 0 -> [_ _ _ _ _ _ _ _]
      event Timeout {
        n56 = event-data() -> ()  [unwired: 1 in, 3 out]
        n57 = local write "Write controls"(FALSE ("manual_reset")) -> ()
      }
      event "Z_OnSwitch": Value Change {
        n58 = event-data() -> ()  [unwired: 1 in, 6 out]
        n59 = local write "Write controls"(TRUE ("manual_reset")) -> ()
      }
      event "Z_Hswitch": Value Change {
        n60 = event-data() -> ()  [unwired: 1 in, 6 out]
        n61 = local write "Write controls"(TRUE ("manual_reset")) -> ()
      }
      event "Y_SP": Value Change {
        n62 = event-data() -> ()  [unwired: 1 in, 6 out]
        n63 = local write "Write controls"(TRUE ("manual_reset")) -> ()
      }
      event "ALRL1_reset": Value Change {
        n64 = event-data() -> ()  [unwired: 1 in, 6 out]
        n65 = local write "Write controls"(TRUE ("manual_reset")) -> ()
      }
      event "ALRL1_reset": Mouse Down {
        n66 = event-data() -> ()  [unwired: 1 in, 8 out]
        n67 = local write "Write controls"(TRUE ("manual_reset")) -> ()
      }
      event "ALRL2_reset": Value Change {
        n68 = event-data() -> ()  [unwired: 1 in, 6 out]
        n69 = local write "Write controls"(TRUE ("manual_reset")) -> ()
      }
      event "ALRL2_reset": Mouse Down {
        n70 = event-data() -> ()  [unwired: 1 in, 8 out]
        n71 = local write "Write controls"(TRUE ("manual_reset")) -> ()
      }
    }
    n72 = Coerce To Type(0:w159, 1:w154) -> (2:w119:T9)
    n73 = Coerce To Type(0:w160, 1:Y_source."initialize" ("Y_Source")) -> (2:w145:T9)
    n74 = Equal?(x=w174, y=w173) -> (x = y?=w124:bool)
    n75 = Coerce To Type(0:w194, 1:w153) -> ()  [unwired: 1 out]
    n76 = Coerce To Type(0:w193, 1:Z_State."on" ("Z_State_heating")) -> (2:w144:T11)
    n77 = Coerce To Type(0:w188, 1:ZM_State."restart_delay" ("ZM_State_heating")) -> (2:w156:T13)
    n78 = call "Is Value Changed.vim"("value"=w132) -> ("changed or first call?"=w141:bool)
    n79 = Bundle By Name(cluster=T10 {"connect"=FALSE, "SP_Source"=enum."initialize", "SP_Set"=0.0, "SP"=0.0} ("source"), "connect"=w124, "SP_Source"=w119, "SP_Set"=w122, "SP"=w122) -> (w131:T10)
    n80 = Bundle By Name(cluster=T12 {"connect"=FALSE, "Z_Source"=enum."initialize", "Z_State_heating"=enum."initialization"} ("source"), "connect"=w124, "Z_Source"=w145, "Z_State_heating"=w144) -> (w143:T12)
    n81 = property on="Z_OnSwitch" class="Z_OnSwitch (strict)"() -> ("timer end"=w149:bool)  [unwired: 2 in, 2 out]
    n82 = Bundle By Name(cluster=cluster{"connect":bool, "Z_Source":T9} {"connect"=FALSE, "Z_Source"=enum."initialize"} ("source"), "connect"=w124, "Z_Source"=w145) -> (w136:cluster{"connect":bool, "Z_Source":T9})
    n83 = property on="Z_Hswitch" class="Z_Hswitch (strict)"() -> ("timer end"=w135:bool)  [unwired: 2 in, 2 out]
    n84 = property on="Y_SP" class="Y (strict)"() -> ("timer end"=w130:bool)  [unwired: 2 in, 2 out]
    n85 = disable-structure shown="Disabled" {
      disable-tunnel: w141 -> [w218 _]
      disable-tunnel: w132 -> [w217 _]
      frame Disabled {
        n86 = case shown="True" w218 {
          tunnel: w217 -> [_ w220]
          frame False {
          }
          frame True {
            w219 = u32 16316664 ("Color Box")
            n87 = Unbundle By Name(w220) -> ("visible"=w221:bool)  [unwired: 1 out]
            n88 = property on="PV" class="Slide (strict)"("Fill Color"=w219) -> ("DigDisps[]"=w224:refnum<vi>[])  [unwired: 2 in, 2 out]
            n89 = Index Array(array=w224, index=0) -> (element=w222:refnum<vi>)
            n90 = property on="Property Node" class="DigNum"(reference=w222, "NumText.BGColor"=w219, "NumText.Visible"=w221) -> ()  [unwired: 1 in, 2 out]
          }
        }
      }
      frame Enabled {
      }
    }
    n91 = local read "name"() -> (w163:string)
    n92 = Not(x=w149) -> (.not. x?=w150:bool)
    n93 = Not(x=w135) -> (.not. x?=w139:bool)
    n94 = Not(x=w130) -> (.not. x?=w128:bool)
    n95 = call "Is Value Changed.vim"("value"=w143) -> ("changed or first call?"=w146:bool)
    n96 = call "Is Value Changed.vim"("value"=w136) -> ("changed or first call?"=w140:bool)
    n97 = call "Is Value Changed.vim"("value"=w131) -> ("changed or first call?"=w129:bool)
    n98 = feedback #1() -> (w151:bool)  [unwired: 1 in]
    n99 = feedback-in #1(w150) -> ()
    n100 = feedback #2() -> (w138:bool)  [unwired: 1 in]
    n101 = feedback-in #2(w139) -> ()
    n102 = feedback #3() -> (w127:bool)  [unwired: 1 in]
    n103 = feedback-in #3(w128) -> ()
    n104 = Unbundle By Name(w133) -> ("Z.ALR  L1"=w148:bool, "Z.ALR  L2"=w147:bool)
    n105 = String Length(string=w163) -> (length=w208:i32)
    n106 = Compound Arithmetic op=OR(w146, w150, w151) -> (w152:bool)
    n107 = Compound Arithmetic op=OR(w140, w139, w138) -> (w137:bool)
    n108 = Compound Arithmetic op=OR(w129, w128, w127) -> (w126:bool)
    n109 = Index Array(array=string[] ["инициализация", "остановлен", "получен сигнал на пуск", "подан сигнал на включение", "разогрев", "нагреватель включен", "получен сигнал на останов нагревателя (задержка перед отключением)", "снижение нагрузки", "снят сигнал на пуск", "охлаждение", "задержка повторного старта"], index=w156) -> (element=w201:string)
    "Z5 State" <- w201
    n110 = Replace Substring(2:3 ("length (len. of substring)"), 3:15 ("offset (0)"), 4:w163, 5:w213) -> (1:w210:string)  [unwired: 1 out]
    n111 = case shown="True" w137 {
      tunnel: w136 -> [_ w226]
      frame False {
      }
      frame True {
        n112 = property on="Z_Hswitch" class="Z_Hswitch (strict)"("State"=w226) -> ()  [unwired: 2 in, 2 out]
      }
    }
    n113 = case shown="True" w126 {
      tunnel: w131 -> [_ w225]
      frame False {
      }
      frame True {
        n114 = property on="Y_SP" class="Y (strict)"("State"=w225) -> ()  [unwired: 2 in, 2 out]
      }
    }
    n115 = case shown="True" w152 {
      tunnel: w143 -> [_ w227]
      frame False {
      }
      frame True {
        n116 = property on="Z_OnSwitch" class="Z_OnSwitch (strict)"("State"=w227) -> ()  [unwired: 2 in, 2 out]
      }
    }
    n117 = call "heating_visu_colors.vi"("Z_State"=w144, "Z_Source"=w145) -> ("N ring"=→"Z3 ind":u16)  [unwired: 6 in, 3 out]
    n118 = property on="ALRL1_reset" class="Bool"("Visible"=w148) -> ()  [unwired: 2 in, 2 out]
    n119 = property on="ALRL2_reset" class="Bool"("Visible"=w147) -> ()  [unwired: 2 in, 2 out]
    n120 = Unbundle("Y_SP") -> (w117:dbl)  [unwired: 2 out]
    n121 = Divide(x=w195, y=u32 1000) -> (x/y=→"T stage":dbl)
    n122 = Compound Arithmetic op=ADD(15 ("offset (0)"), w208, 2 ("value")) -> (w206:i32)
    n123 = Replace Substring(2:66 ("value"), 3:w206, 4:w201, 5:w210) -> (1:w205:string)  [unwired: 1 out]
    n124 = Boolean To (0,1)(Boolean="Z_Hswitch") -> (0, 1=w197:i16)
    n125 = Boolean To (0,1)(Boolean="Z_Hswitch") -> (0, 1=w192:i16)
    n126 = Select(t=Z_State."on" ("Z_State"), s="Z_OnSwitch", f=Z_State."stop ready" ("Z_State")) -> (s? t:f=w200:T11)
    n127 = Select(t=Y_state."auto" ("Y_HSetState"), s="Z_Hswitch", f=Y_state."hand" ("Y_HSetState")) -> (s? t:f=w189:T16)
    n128 = Or(x="ALRL1_reset", y="ALRL2_reset") -> (x .or. y?=w185:bool)
    n129 = property on="Z3 ind" class="Ring (strict)"("TipStrip"=w205) -> ()  [unwired: 2 in, 2 out]
    n130 = Bundle By Name(cluster=T15 {"Z_HSw"=0, "Z_HSetState"=0, "Y_HSw"=0, "Y_HSetState"=0, "SP"=0.0, "Y_H"=0.0, "Reset_ALR"=FALSE} ("HT1_in"), "Z_HSw"=w197, "Z_HSetState"=w200, "Y_HSw"=w192, "Y_HSetState"=w189, "SP"=50.0, "Y_H"=w117, "Reset_ALR"=w185) -> (w172:T15)
    n131 = case shown="True" "Write controls" {
      tunnel: w172 -> [_ w246]
      tunnel: w171 -> [w236 w238]
      tunnel: w169 -> [_ w242]
      tunnel: w168 -> [_ w244]
      tunnel: [w236 w240] -> w167
      frame False {
      }
      frame True {
        n132 = Flatten To JSON(anything=w246, error in (no error)=w238) -> (JSON string=w239:string, 11:w237:errorcluster)  [unwired: 1 in]
        n133 = Get Date/Time In Seconds() -> (seconds since 1Jan1904=w245:timestamp)
        n134 = call "Write element.vi"("seconds since 1Jan1904"=w245, "Variant"=w239, "request in"=w244) -> ("request out"=w243:T4)  [unwired: 8 in]
        n135 = Build Array(w243) -> (w241:T4[])
        n136 = call-poly <vilib>:"Multiple Write.vi"("error in (no error)"=w237, "requests"=w241, "OPC UA client refnum in"=w242) -> ("error out"=w240:errorcluster)  [unwired: 5 in, 3 out]
      }
    }
    n137 = control-ref of="This VI"() -> (w180:refnum<vi>)
    "This VI" <- w180
    n138 = disable-structure shown="Disabled" {
      frame Disabled {
      }
      frame Enabled {
      }
    }
    n139 = Wait (ms)(milliseconds to wait=u32 100) -> ()  [unwired: 1 out]
    n140 = global read "Global stop.vi" "Stop"() -> (w183:bool)
    n141 = Compound Arithmetic op=OR(w167, w183, "stop") -> (w166:bool)
    n142 = case shown="True" w166 {
      tunnel: w165 -> [_ w248]
      tunnel: [_ w247] -> w164
      frame False {
      }
      frame True {
        n143 = call <vilib>:"Send Local Message.vi"("message queue in"=w248, "message name"="Exit") -> ("error out"=w247:errorcluster)  [unwired: 11 in, 2 out]
      }
    }
  }
  n144 = Merge Errors(w11, w13) -> (w25:errorcluster)
  n145 = disable-structure shown="Disabled" {
    disable-tunnel: w38 -> [w250 _]
    frame Disabled {
      n146 = invoke class="VI" method="FP.Close"(reference=w250) -> ()  [unwired: 2 in, 3 out]
    }
    frame Enabled {
    }
  }
  n147 = call <vilib>:"Delete Monitored Nodes.vi"("error in (no error)"=w25, "node IDs"=w10, "subscription ID in"=w24, "OPC UA client refnum in"=w12) -> ("error out"=w29:errorcluster, "OPC UA client refnum out"=w30:T7)  [unwired: 3 in, 3 out]
  n148 = Build Array(w24) -> (w26:T8[])
  n149 = call <vilib>:"Delete Subscriptions.vi"("error in (no error)"=w29, "subscription IDs"=w26, "OPC UA client refnum in"=w30) -> ("error out"=w27:errorcluster, "OPC UA client refnum out"=w28:T7)  [unwired: 6 in, 1 out]
  n150 = call <vilib>:"Disconnect.vi"("error in (no error)"=w27, "OPC UA client refnum in"=w28) -> ("error out"=w5:errorcluster)  [unwired: 9 in]
  n151 = Merge Errors(w5, w4) -> (→"error out":errorcluster)
